vi "RP Read Subset TCP.vi"(4 "Logic tag":u16, 6 "Bytes per sample":i32, 7 "Samples per trigger increment":i32=2, 8 "Error In":errorcluster, 9 "Post-trigger samples":u64=11534336 format="0x%x (%d)", 10 "Pre-trigger samples":i32=-100000 format="0x%x (%d)", 11 "connection ID":refnum<k5>) -> (0 "Error Out":errorcluster, 1 "Record start pos":u32=1, 2 "Data stream":string, 3 "connection ID out":refnum<k5>)   [LabVIEW 2025]
uses:
  RP Command.ctl
  RP Status Offsets.ctl
panel:
  out "size in":i32[](array[numeric])
  out "size out":i32[](array[numeric])
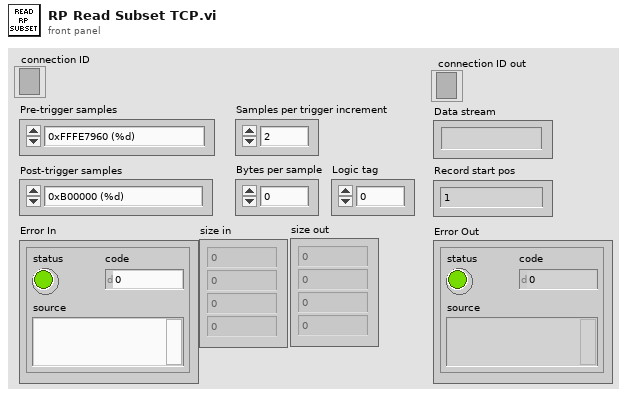
[diagram p1: front panel]
types:
  T1 = typedef "RP Status Offsets.ctl" = u16
  T2 = typedef "RP Command.ctl" = enum16{"Reset", "Read IDN", "Stop server", "Get status", "Get temperature", "Connect client", "Arm", "Software trigger", "Get whole buffer", "Get chunk", "System call", "Get config", "Set config", "Recieve data", "Recieve Calibartion", "Transmit data"}
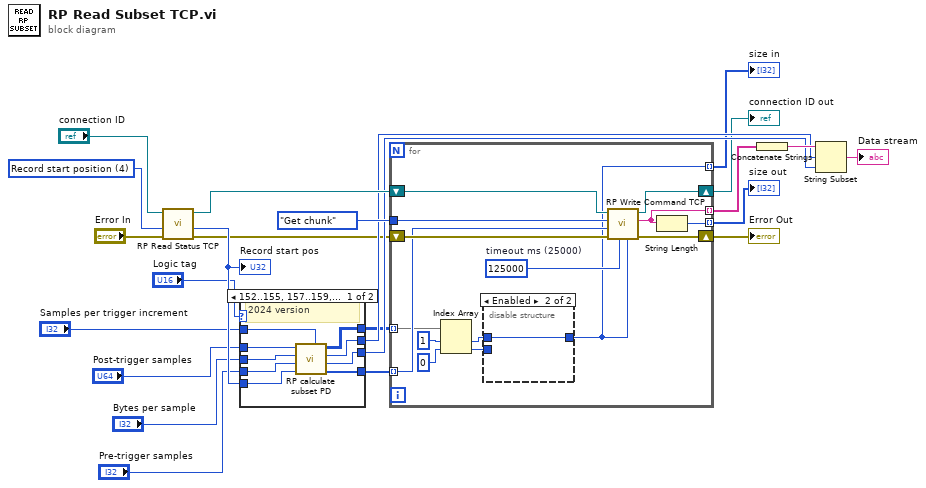
[diagram p0: block diagram]
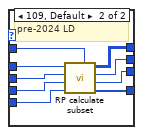
[diagram p2: hidden frame]
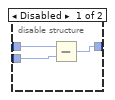
[diagram p3: hidden frame]
diagram:
  w22 = T1 4 items=["Writer address"=0, "Record start position"=4, "Trig state etc."=8, "RxFIFO counter"=24, "TxFIFO counter"=28] ("Status offset")
  n1 = call "RP Read Status TCP.vi"("Error In"="Error In", "Status offset"=w22, "connection ID"="connection ID") -> ("Error Out"=w12:errorcluster, "Status response"=w21:u32, "connection ID out"=w20:refnum<k5>)  [unwired: 6 in]
  "Record start pos" <- w21
  n2 = case shown="152..155, 157..159, 164, 169" "Logic tag" {
    tunnel: w21 -> [w28 w41]
    tunnel: [w26 w40] -> w19
    tunnel: [w25 w39] -> w16
    tunnel: [w24 w38] -> w15
    tunnel: [w27 w37] -> w8
    tunnel: "Samples per trigger increment" -> [w32 w36]
    tunnel: "Bytes per sample" -> [w30 w35]
    tunnel: "Post-trigger samples" -> [w31 w34]
    tunnel: "Pre-trigger samples" -> [w29 w33]
    frame 152..155, 157..159, 164, 169 {
      # "2024 version"
      n3 = call "RP calculate subset PD.vi"("Samples per trigger increment"=w32, "Trigger start position"=w28, "Pre-trigger samples"=w29, "Bytes per sample"=w30, "Post-trigger samples"=w31) -> ("Merged subsets"=w26:u64[], "record length"=w24:i32, "pre-trigger trim"=w25:i32, "Subsets"=w27:i32[][])  [unwired: 3 in]
    }
    frame 109, Default {
      # "pre-2024 LD"
      n4 = call "RP calculate subset.vi"("Samples per trigger increment"=w36, "Trigger start position"=w41, "Pre-trigger samples"=w33, "Bytes per sample"=w35, "Post-trigger samples"=w34) -> ("Merged subsets"=w40:u64[], "record length"=w38:i32, "pre-trigger trim"=w39:i32, "Subsets"=w37:i32[][])  [unwired: 3 in]
    }
  }
  n5 = for {
    tunnel: RP_Command."Get chunk" ("Command number") -> [w56]
    shift-right: [w45] -> w10
    shift-left: w12 -> [w55]
    shift-right: [w44] -> w13
    shift-left: w20 -> [w54]
    tunnel: w19 -> [w53] mode=indexing
    tunnel: [w43] -> w18 mode=indexing
    tunnel: w8 -> [w51] mode=indexing
    tunnel: [w47] -> w3 mode=indexing
    tunnel: [w42] -> w2 mode=indexing
    w46 = 125000  # timeout ms (25000)
    n6 = Index Array(array=w51, index #1=1 ("index"), index #2=0 ("index")) -> (element #1=w50:i32, element #2=w49:i32)
    n7 = disable-structure shown="Enabled" {
      disable-tunnel: w50 -> [w59 w60]
      disable-tunnel: w49 -> [w58 _]
      disable-tunnel: [w57 w60] -> w42
      frame Disabled {
        n8 = Subtract(x=w59, y=w58) -> (x-y=w57:i32)
      }
      frame Enabled {
      }
    }
    n9 = call "RP Write Command TCP.vi"("bytes to read"=w42, "timeout ms (25000)"=w46, "Error In"=w55, "Command payload"=w53, "Command number"=w56, "connection ID"=w54) -> ("Error Out"=w45:errorcluster, "data out"=w43:string, "connection ID out"=w44:refnum<k5>)  [unwired: 2 in, 1 out]
    n10 = String Length(string=w43) -> (length=w47:i32)
  }
  "connection ID out" <- w13
  "Error Out" <- w10
  "size out" <- w3
  "size in" <- w2
  n11 = Concatenate Strings(w18) -> (w17:string)
  n12 = String Subset(string=w17, offset (0)=w16, length (rest)=w15) -> (substring=→"Data stream":string)
